vi "GetSystemDefinitionNodeByName.vi"(8 "error in (no error)":errorcluster, 10 "nodepath":string, 11 "SystemDefinition in":refnum<k39>) -> (0 "error out":errorcluster, 2 "BaseNodeType":refnum<k39>, 3 "SystemDefinition out":refnum<k39>)   [LabVIEW 2027, in "VeriStandTestUtilities.lvlib"]
uses:
  VeriStandTestUtilities.lvlib
  C:/NetCoreDLL/NationalInstruments.VeriStand.SystemDefinitionAPI.dll
  NetCoreDLL/NationalInstruments.VeriStand.SystemDefinitionAPI.dll
  C:/NetCoreDLL/NationalInstruments.VeriStand.SystemStorage.dll
  NetCoreDLL/NationalInstruments.VeriStand.SystemStorage.dll
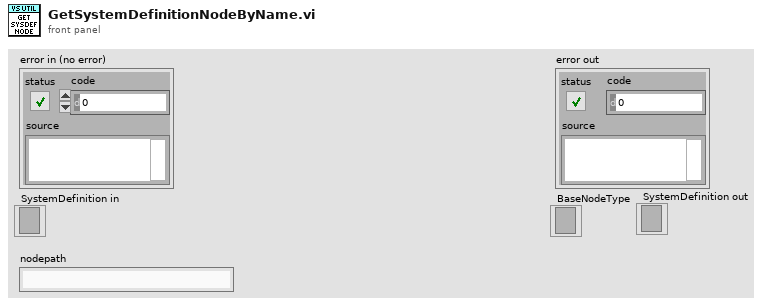
[diagram p1: front panel]
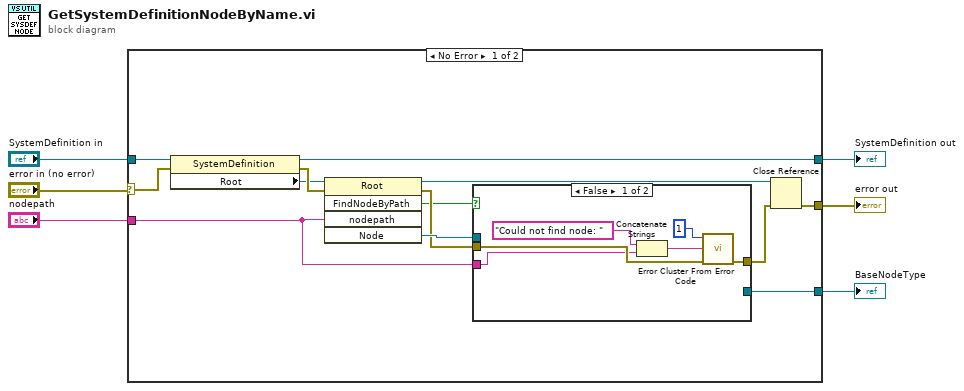
[diagram p0: block diagram]
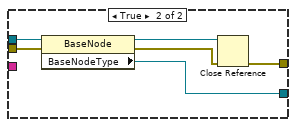
[diagram p2: hidden frame]
diagram:
  n1 = case shown="No Error" "error in (no error)" {
    selector: "error in (no error)" -> [w18 w33]
    tunnel: "SystemDefinition in" -> [w19 w32]
    tunnel: "nodepath" -> [w9 _]
    tunnel: [w10 _] -> w2
    tunnel: [w8 w33] -> w3
    tunnel: [w7 w32] -> w1
    frame No Error {
      n2 = property class="SystemDefinition"(reference=w19, error in=w18) -> (reference out=w7:refnum<k39>, error out=w17:errorcluster, "Root"=w16:refnum<k39>)
      n3 = invoke class="Root" method="FindNodeByPath"(reference=w16, error in=w17, "nodepath"=w9) -> (reference out=w15:refnum<k39>, error out=w13:errorcluster, "FindNodeByPath"=w11:bool, "Node"=w14:refnum<k39>)  [unwired: 2 in, 1 out]
      n4 = case shown="False" w11 {
        tunnel: w14 -> [_ w31]
        tunnel: w13 -> [w25 w30]
        tunnel: [w24 w26] -> w12
        tunnel: [_ w29] -> w10
        tunnel: w9 -> [w21 _]
        frame False {
          n5 = Concatenate Strings("Could not find node: " ("error message (\"\")"), w21) -> (w20:string)
          n6 = call <vilib>:"Error Cluster From Error Code.vi"("error in (no error)"=w25, "error message (\"\")"=w20, "error code (0)"=1) -> ("error out"=w24:errorcluster)  [unwired: 6 in]
        }
        frame True {
          n7 = property class="BaseNode"(reference=w31, error in=w30) -> (reference out=w28:refnum<k39>, error out=w27:errorcluster, "BaseNodeType"=w29:refnum<k39>)
          n8 = Close Reference(reference=w28, error in (no error)=w27) -> (error out=w26:errorcluster)
        }
      }
      n9 = Close Reference(reference=w15, error in (no error)=w12) -> (error out=w8:errorcluster)
    }
    frame Error {
    }
  }
  "error out" <- w3
  "BaseNodeType" <- w2
  "SystemDefinition out" <- w1
